vi "Create.vi"(8 "error in (no error)":errorcluster) -> (0 "error out":errorcluster, 3 "GA-Extend-Cmd out":refnum<class "GA-Extend-Cmd.lvclass">)   [LabVIEW 2013, in "GA-Extend-Cmd.lvclass"]
uses:
  GA-Extend-Cmd.lvclass
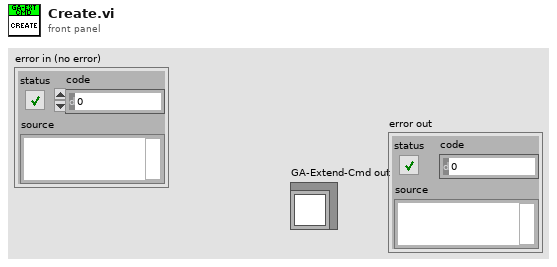
[diagram p1: front panel]
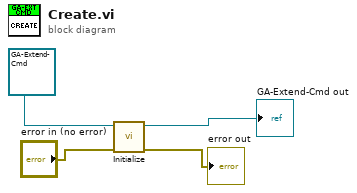
[diagram p0: block diagram]
diagram:
  n1 = call-dynamic "Initialize.vi"("error in (no error)"="error in (no error)", "GA-Extend-Cmd in"=refnum<class "GA-Extend-Cmd.lvclass"> refnum ("GA-Extend-Cmd.lvclass")) -> ("error out"=→"error out":errorcluster, "GA-Extend-Cmd out"=→"GA-Extend-Cmd out":refnum<class "GA-Extend-Cmd.lvclass">)  [unwired: 8 in]
